vi "GetSmplDepth.vi"(8 "错误输入（无错误）":errorcluster, 11 "Chan":u8) -> (0 "错误输出":errorcluster, 3 "返回值":u16)   [LabVIEW 2018]
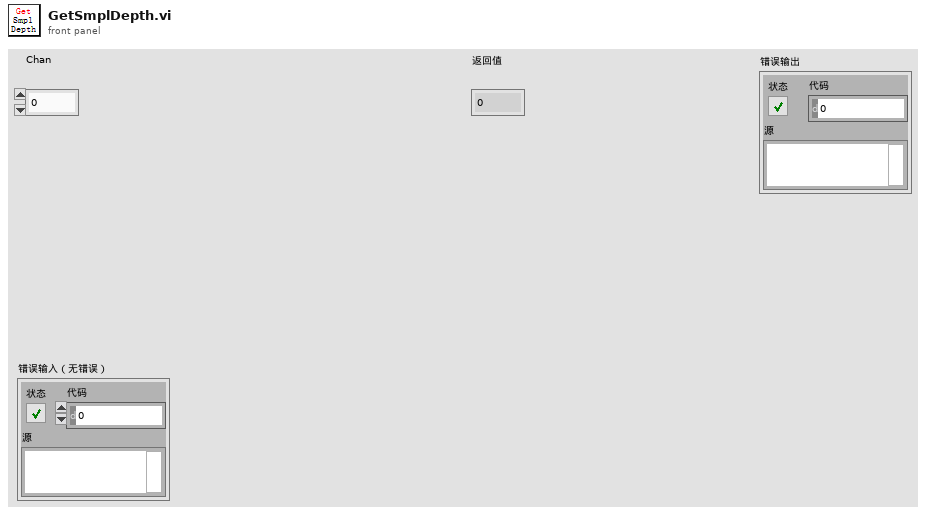
[diagram p1: front panel]
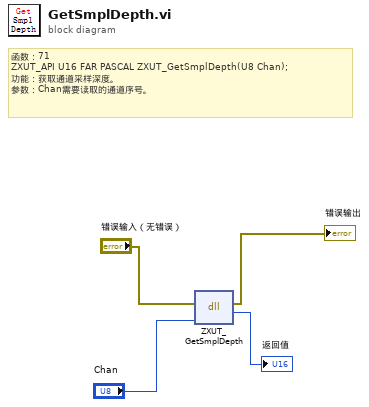
[diagram p0: block diagram]
diagram:
  # "函数：71\nZXUT_API U16\tFAR PASCAL ZXUT_GetSmplDepth(U8 Chan);\n功能：获取通道采样深度。\n参数：Chan需要读取的通道序号。"
  n1 = dll-call lib="PTH2Rabs E软件项目超声超声子VI函数VI\tTCG处理ZXUTConfigMgr.dll" fn="ZXUT_GetSmplDepth"(error in="错误输入（无错误）", "Chan"="Chan") -> (error out=→"错误输出":errorcluster, "返回值"=→"返回值":u16)  [unwired: 3 in, 1 out]
